vi "Cryostat JSON.vi"(11 "Instrument.Cryostat in":refnum<class "Instrument.Cryostat.lvclass">) -> ()   [LabVIEW 2019, in "Instrument.Cryostat.lvclass"]
uses:
  Instrument.Cryostat.lvclass
  Typedefs/Magnet Mode--Enum.ctl
  Typedefs/Magnet Axis--Enum.ctl
  Typedefs/setMagnet--cluster.ctl
  Typedefs/Rotator Axis--Enum.ctl
  Typedefs/setAngle--cluster.ctl
  Typedefs/setTemperature--cluster.ctl
  <vilib>/PRIrvin/JSON-RPC/JSON-RPC.lvlib
  <vilib>/JDP Science/JSONtext/JSONtext.lvlib
  4589dab0-be73-4d70-a91b-5f3eda8b291f.vi
panel:
  out "$Paths":string[](array[string])
  out "<JSON> Items":string[](array[string]) caption="<JSON>Items"
  out "Names":string[](array[string])
  out "Params":string[](array[string])
  out "JSON-RPC":string
  out "Data":dbl
  out "Data out":T1={"field"=0.0, "rate"=0.0, "axis"=enum."Z", "mode"=enum."Persistent"}
  out "error out":errorcluster
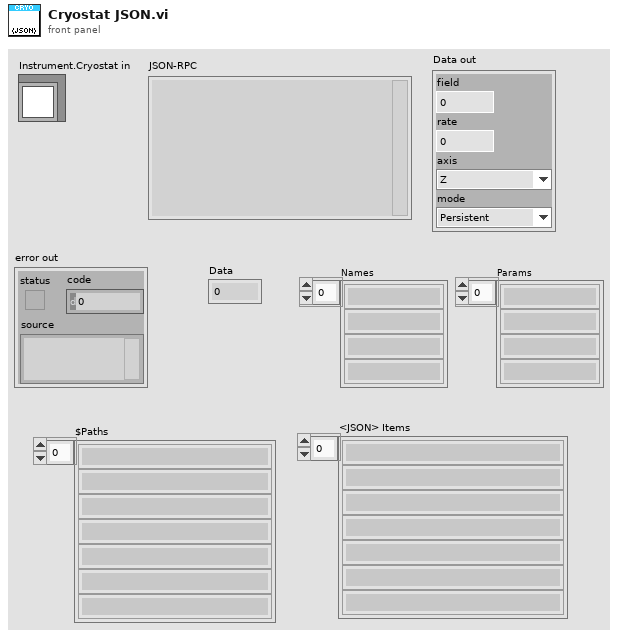
[diagram p1: front panel]
types:
  T1 = typedef "Instrument.Cryostat.lvclass/setMagnet--cluster.ctl" = cluster{"field":dbl, "rate":dbl, "axis":T2, "mode":T3}
  T2 = typedef "Instrument.Cryostat.lvclass/Magnet Axis--Enum.ctl" = enum16{"X", "Y", "Z"}
  T3 = typedef "Instrument.Cryostat.lvclass/Magnet Mode--Enum.ctl" = enum16{"Persistent", "Driven"}
  T4 = typedef "Instrument.Cryostat.lvclass/setTemperature--cluster.ctl" = cluster{"temperature":dbl, "rate":dbl, "channel":i32}
  T5 = typedef "Instrument.Cryostat.lvclass/setAngle--cluster.ctl" = cluster{"angle":dbl, "rate":dbl, "channel":i32}
  T6 = typedef "Instrument.Cryostat.lvclass/Rotator Axis--Enum.ctl" = enum16{"Axis 1", "Axis 2"}
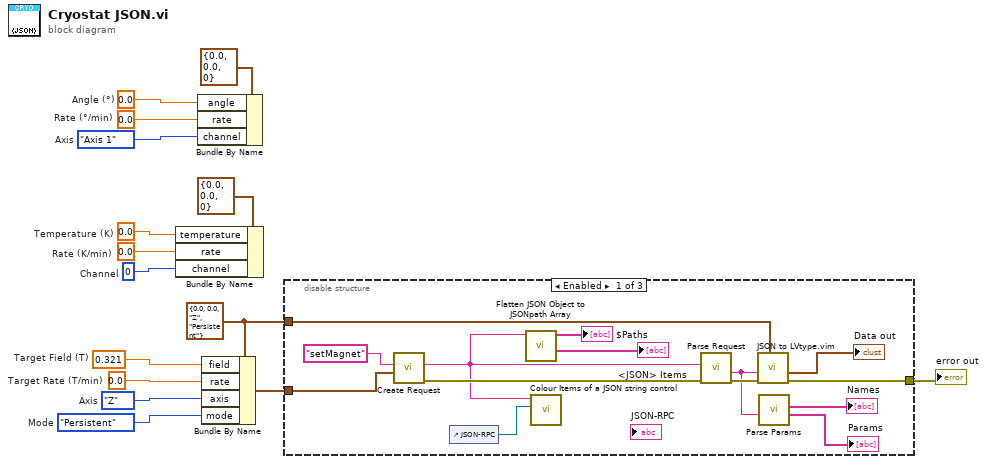
[diagram p0: block diagram]
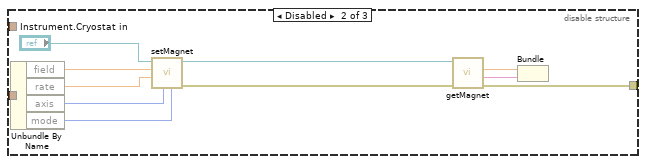
[diagram p2: hidden frame]
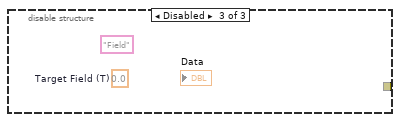
[diagram p3: hidden frame]
diagram:
  w6 = 0  # Channel
  w12 = 0.0  # Rate (K/min)
  w5 = 0.0  # Temperature (K)
  w14 = 0.0  # Rate (°/min)
  w3 = Rotator_Axis--Enum."Axis 1"  # Axis
  w4 = 0.0  # Angle (°)
  w1 = T1 {"field"=0.0, "rate"=0.0, "axis"=enum."Z", "mode"=enum."Persistent"} ("output cluster")
  w7 = 0.321  # Target Field (T)
  w8 = 0.0  # Target Rate (T/min)
  w9 = Magnet_Axis--Enum."Z"  # Axis
  w10 = Magnet_Mode--Enum."Persistent"  # Mode
  n1 = Bundle By Name(cluster=T4 {"temperature"=0.0, "rate"=0.0, "channel"=0}, "temperature"=w5, "rate"=w12, "channel"=w6) -> ()  [unwired: 1 out]
  n2 = Bundle By Name(cluster=T5 {"angle"=0.0, "rate"=0.0, "channel"=0} ("output cluster"), "angle"=w4, "rate"=w14, "channel"=w3) -> ()  [unwired: 1 out]
  n3 = Bundle By Name(cluster=w1, "field"=w7, "rate"=w8, "axis"=w9, "mode"=w10) -> (w2:T1)
  n4 = disable-structure shown="Enabled" {
    disable-tunnel: [w16 w38 w41] -> w15
    disable-tunnel: w2 -> [w21 w30 _]
    disable-tunnel: w1 -> [w29 _ _]
    frame Enabled {
      n5 = call <vilib>:"Create Request.vi"("params"=w21, "method"="setMagnet") -> ("error out"=w28:errorcluster, "<JSON> Requests"=w22:string)  [unwired: 7 in, 1 out]
      n6 = control-ref of="JSON-RPC"() -> (w25:refnum<vi>)
      n7 = call <vilib>:"Flatten JSON Object to JSONpath Array.vi"("JSON"=w22) -> ("<JSON>"=→"<JSON> Items":string[], "$Paths"=→"$Paths":string[])  [unwired: 8 in, 1 out]
      n8 = call <vilib>:"Colour Items of a JSON string control.vi"("String Control"=w25, "JSON"=w22) -> ()  [unwired: 9 in, 1 out]
      n9 = call <vilib>:"Parse Request.vi"("error in (no error)"=w28, "<JSON> Requests"=w22) -> ("error out"=w19:errorcluster, "Params"=w18:string)  [unwired: 6 in, 2 out]
      n10 = call "JSON to LVtype.vim"("type"=w29, "error in (no error)"=w19, "JSON Data in"=w18) -> ("error out"=w16:errorcluster, "Data out"=→"Data out":T1)  [unwired: 7 in]
      n11 = call <vilib>:"Parse Params.vi"("<JSON> Params"=w18) -> ("Params"=→"Params":string[], "Names"=→"Names":string[])  [unwired: 8 in, 1 out]
    }
    frame Disabled {
      n12 = Unbundle By Name(w30) -> ("field"=w37:dbl, "rate"=w36:dbl, "axis"=w35:T2, "mode"=w34:T3)
      n13 = call-dynamic "setMagnet.vi"("Mode"=w34, "Axis"=w35, "Target Rate (T/min)"=w36, "Target Field (T)"=w37, "Instrument.Cryostat in"="Instrument.Cryostat in") -> ("error out"=w32:errorcluster, "Instrument.Cryostat out"=w33:refnum<class "Instrument.Cryostat.lvclass">)  [unwired: 5 in]
      n14 = call-dynamic "getMagnet.vi"("error in (no error)"=w32, "Instrument.Cryostat in"=w33) -> ("error out"=w38:errorcluster, "Status"=w39:string, "B Field (T)"=w40:dbl)  [unwired: 5 in, 2 out]
      n15 = Bundle("B Field (T)"=w40, "Status"=w39) -> ()  [unwired: 1 in, 1 out]
    }
    frame Disabled {
      (unwired) 0.0  # Target Field (T)
      (unwired) "Field" ("$Path or Item Name")
    }
  }
  "error out" <- w15
